vi "X10468 SLM Engine.vi"(0 "Notifier Name":string, 11 "SLM Config Info":string[](array[string])) -> ()   [LabVIEW 2018]
uses:
  X10468 Controls/X10468 SLM Notifier.ctl
  X10468 Controls/X10468 SLM Actions.ctl
  <vilib>/vision/Image Controls.llb/IMAQ Image.ctl
  X10468 Controls/X10468 SLM Last Used.ctl
panel:
  out "Holo Max":dbl
  out "Holo Min":dbl
  out "Flat File":path
  out "SLM Display":T1(plugin-control)
  out "SLM Min":u8
  out "SLM Max":u8
  in  "Mode Amounts":dbl[](array[numeric])
  in  "Holo XY Position":i32[](array[numeric])
  in  "Top Hat Radius":dbl
  in  "Holo Size (px)":i32=10 min=10 max=1000
  in  "Set Flat":bool
  in  "Flat":bool
  in  "Top Hat":bool
  in  "Vortex Direction":bool
  in  "Vortex":bool
  in  "Number of Modes":i32=1 min=1 max=32
  out "Last Error":errorcluster
  in  "Quit":bool
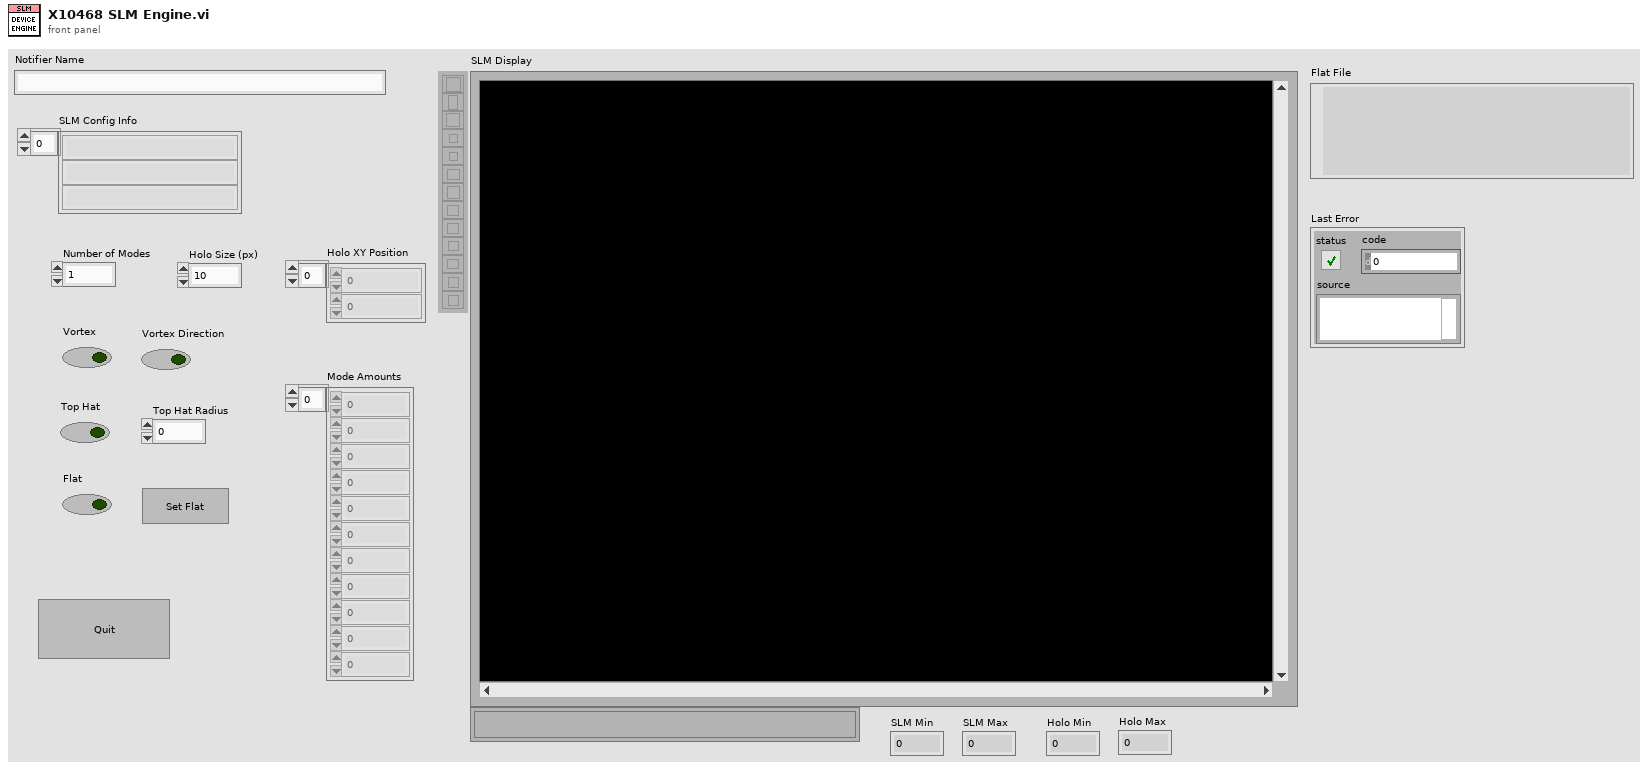
[diagram p1: front panel]
types:
  T1 = typedef "IMAQ Image.ctl" = refnum<image>
  T2 = typedef "X10468 SLM Last Used.ctl" = cluster{"Flat On?":bool, "Vortex On?":bool, "Top Hat On?":bool, "Mode Amps":dbl[], "Number of Modes":i32, "Holo Diameter (px)":i32, "Top Hat Radius":dbl, "Holo Position":i32[], "Flat File Path":string}
  T3 = typedef "X10468 SLM Actions.ctl" = enum16{"Exit Loop", "Get Settings", "Set Flat File", "Change Holo Size", "Change Num Modes", "Change Holo Position", "Change Top Hat Size", "Change Vortex Direction", "Change Mode Amounts", "Flat On/Off", "Vortex On/Off", "Top Hat On/Off", "Make Hologram", "Update SLM Display", "Quit"}
  T4 = typedef "X10468 SLM Notifier.ctl" = cluster{"SLM Actions":T3, "SLM Image":T1, "Flat On?":bool, "Vortex On?":bool, "Top Hat On?":bool, "Mode Amps":dbl[], "Number of Modes":i32, "Holo Diameter (px)":i32, "Top Hat Radius":dbl, "Holo Position":i32[], "Received?":bool, "Flat File Path":path}
  T5 = typedef "Image Type" = u32
  T6 = typedef "LVAllMonitorsDisplayTypeDef.ctl" = cluster{"Bounds":cluster{"Left":i16, "Top":i16, "Right":i16, "Bottom":i16}, "Depth":i16}[]
  T7 = cluster{"Bounds":cluster{"Left":i16, "Top":i16, "Right":i16, "Bottom":i16}, "Depth":i16}
  T8 = enum32{"Invalid", "Standard", "Closed", "Hidden", "Minimized", "Maximized"}
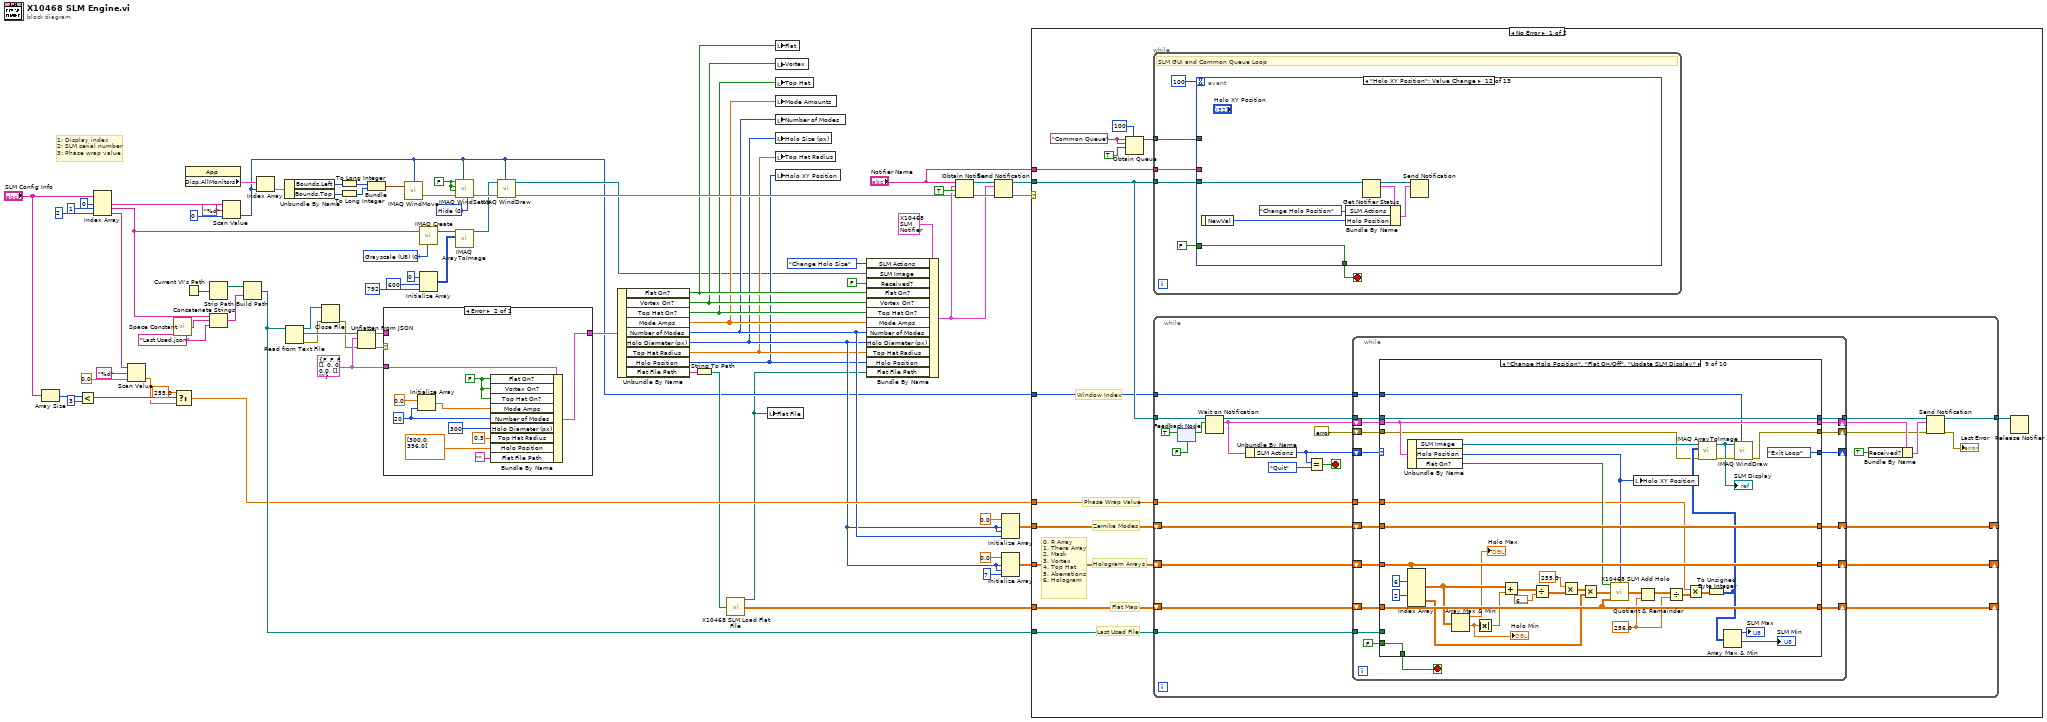
[diagram p0: block diagram]
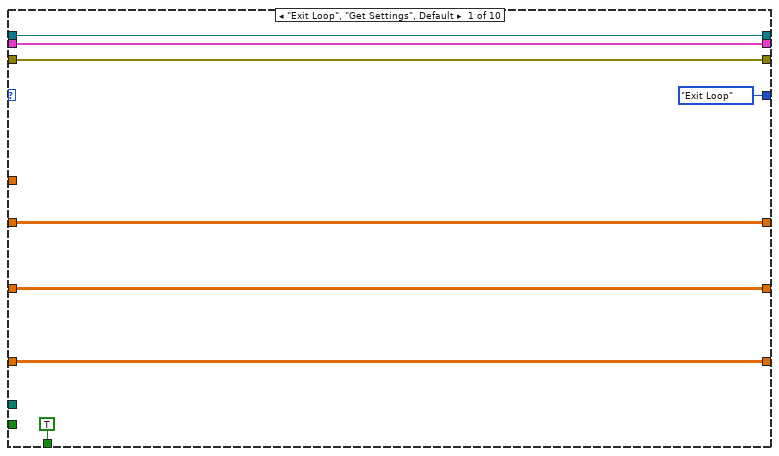
[diagram p3: hidden frame]
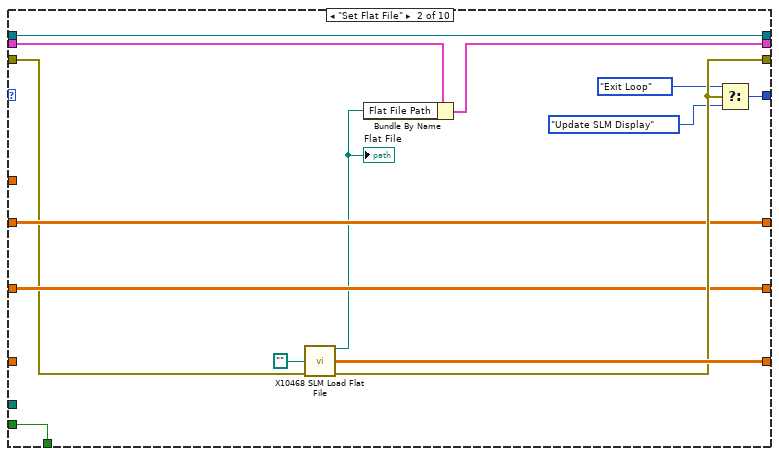
[diagram p4: hidden frame]
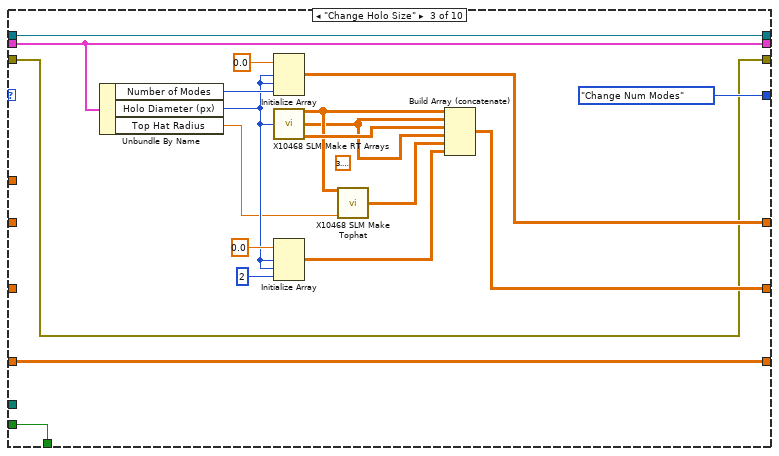
[diagram p5: hidden frame]
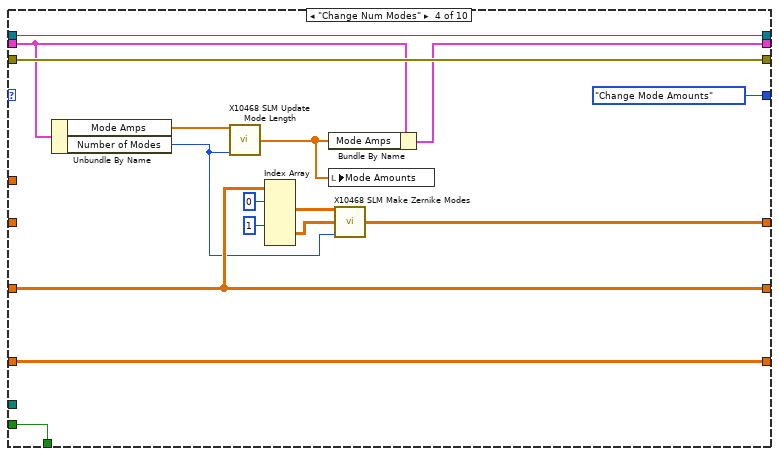
[diagram p6: hidden frame]
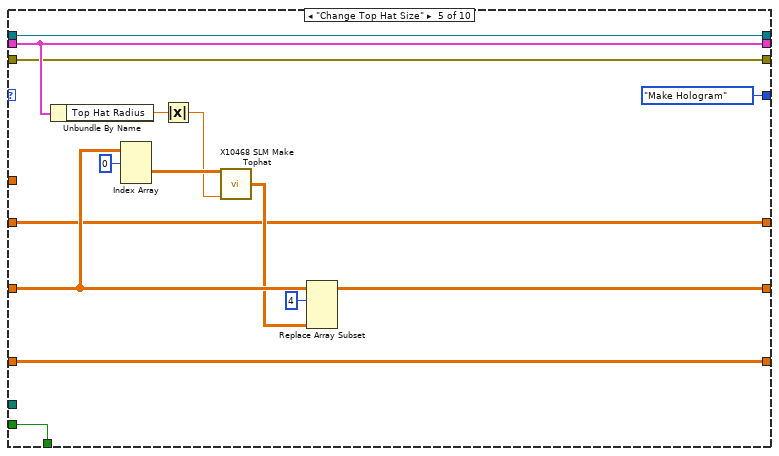
[diagram p7: hidden frame]
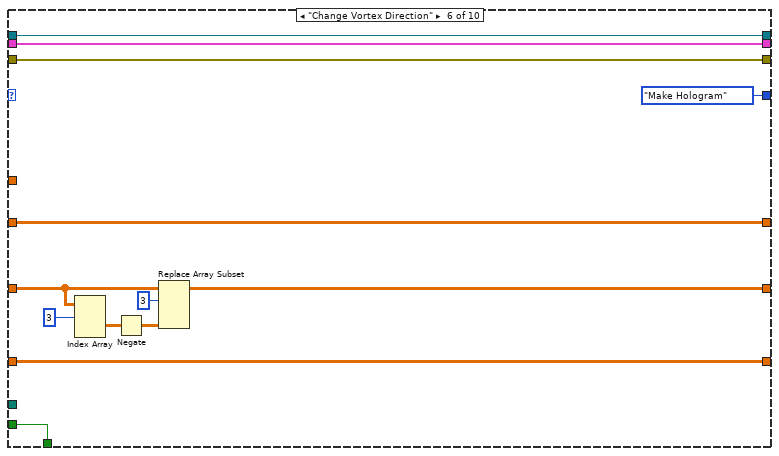
[diagram p8: hidden frame]
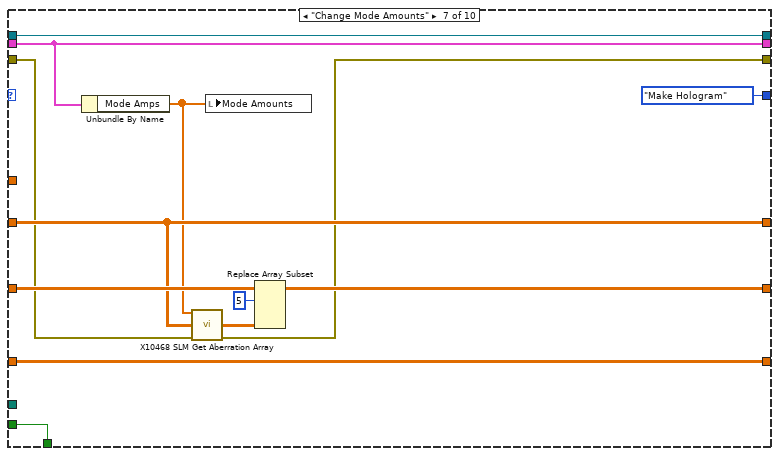
[diagram p9: hidden frame]
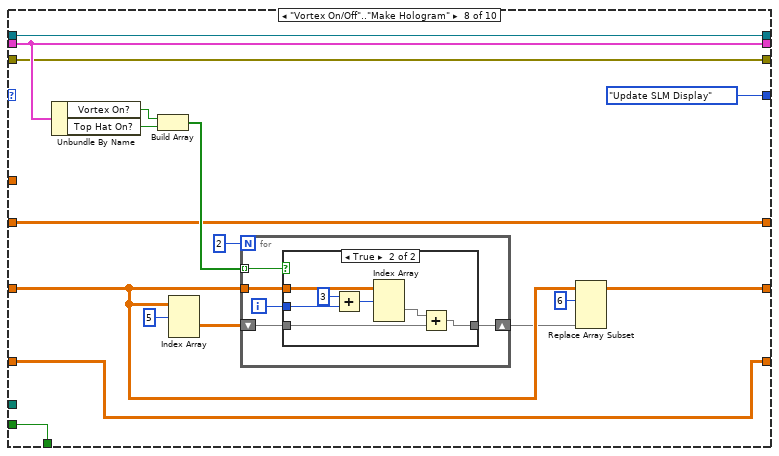
[diagram p10: hidden frame]
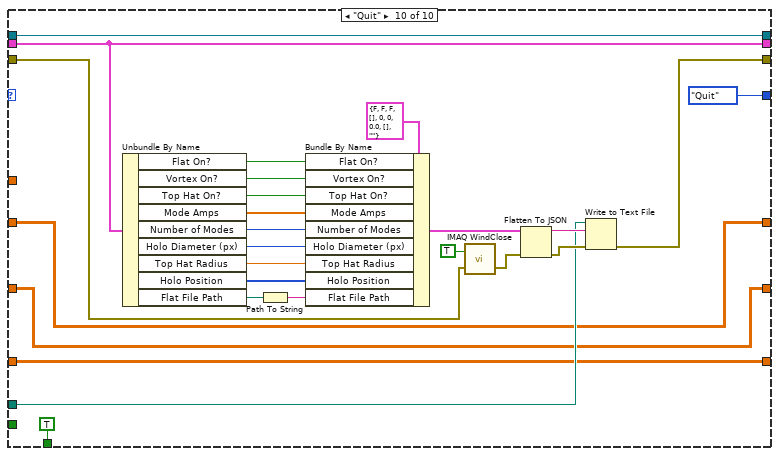
[diagram p12: hidden frame]
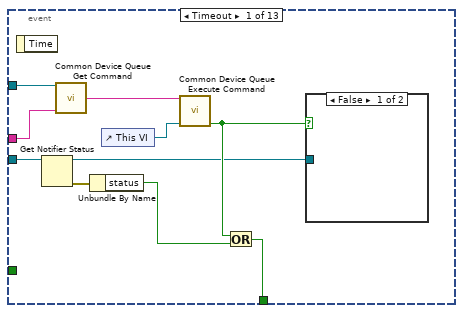
[diagram p13: hidden frame]
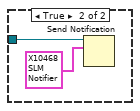
[diagram p14: hidden frame]
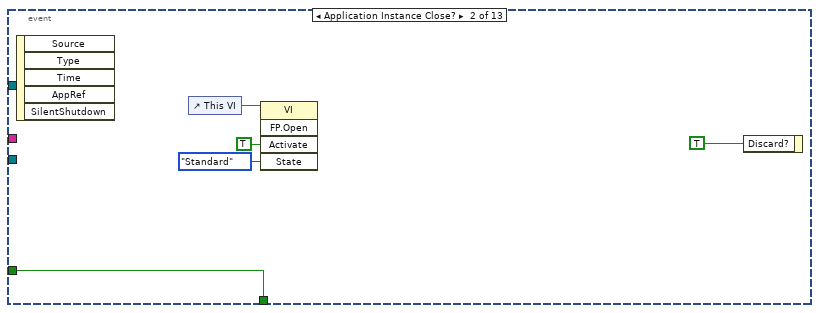
[diagram p15: hidden frame]
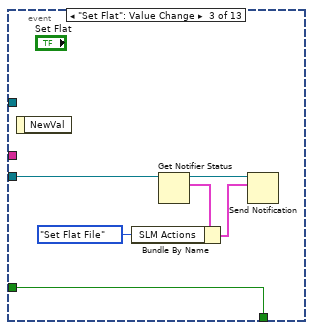
[diagram p16: hidden frame]
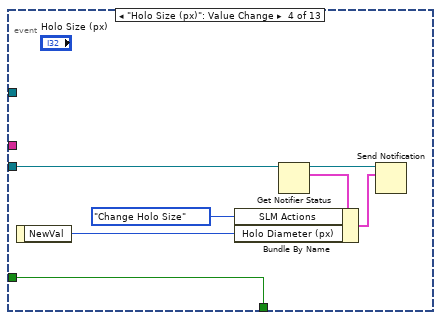
[diagram p17: hidden frame]
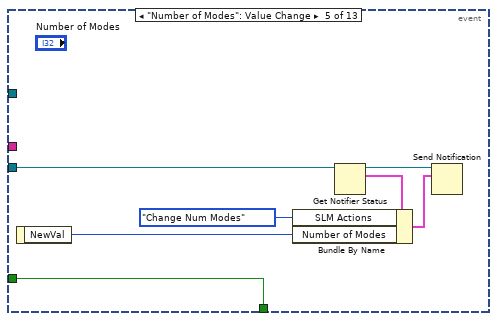
[diagram p18: hidden frame]
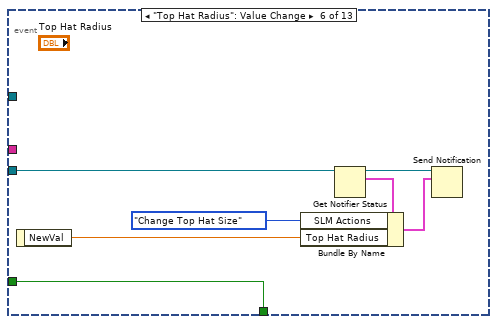
[diagram p19: hidden frame]
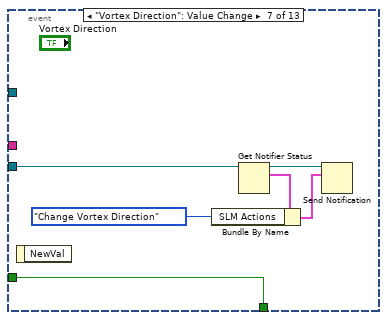
[diagram p20: hidden frame]
diagram:
  w31 = T2 {"Flat On?"=FALSE, "Vortex On?"=FALSE, "Top Hat On?"=FALSE, "Mode Amps"=[], "Number of Modes"=0, "Holo Diameter (px)"=0, "Top Hat Radius"=0.0, "Holo Position"=[], "Flat File Path"=""} ("SLM Notifier")
  w63 = 0 items=["Hide", "Show", "No change"] ("Scrollbars (No change)")
  w64 = FALSE ("Window can grow? (Yes)")
  w78 = T5 0 items=["Grayscale (U8)", "Grayscale (I16)", "Grayscale (SGL)", "Complex (CSG)", "RGB (U32)", "HSL (U32)", "RGB (U64)", "Grayscale (U16)"] ("Image Type")
  # "1: Display index\n2: SLM serial number\n3: Phase wrap value"
  n1 = Array Size(array="SLM Config Info") -> (size(s)=w43:i32)
  n2 = Less?(x=w43, y=3) -> (x < y?=w41:bool)
  n3 = Index Array(array="SLM Config Info", index #1=0 ("index"), index #2=1 ("index"), index #3=2 ("index")) -> (element #1=w72:string, element #2=w38:string, element #3=w45:string)
  n4 = Scan Value(string=w45, format string="%d", default (0 dbl)=0.0) -> (value=w40:dbl)  [unwired: 1 out]
  n5 = call <vilib>:"Space Constant.vi"() -> ("String"=w37:string)
  n6 = Select(t=255.0, s=w41, f=w40) -> (s? t:f=w23:dbl)
  n7 = property class="App"() -> ("Disp.AllMonitors"=w69:T6)  [unwired: 2 in, 2 out]
  n8 = Current VI's Path() -> (path=w75:path)
  n9 = Strip Path(path=w75) -> (stripped path=w74:path)  [unwired: 1 out]
  n10 = Concatenate Strings(w38, w37, "Last Used.json" ("string")) -> (w35:string)
  n11 = Scan Value(string=w72, format string="%d", default (0 dbl)=0) -> (value=w2:i32)  [unwired: 1 out]
  n12 = Build Path(base path=w74, name or relative path=w35) -> (appended path=w24:path)
  n13 = Index Array(array=w69, index=w2) -> (element=w68:T7)
  n14 = Unbundle By Name(w68) -> ("Bounds.Left"=w67:i16, "Bounds.Top"=w27:i16)
  n15 = Read from Text File(file (use dialog)=w24) -> (refnum out=w17:refnum<file>, text=w34:string, error out=w16:errorcluster)  [unwired: 3 in, 1 out]
  n16 = Close File(refnum=w17, error in=w16) -> (error out=w15:errorcluster)  [unwired: 1 out]
  n17 = To Long Integer(number=w27) -> (32bit integer=w26:i32)
  n18 = To Long Integer(number=w67) -> (32bit integer=w66:i32)
  n19 = Unflatten From JSON(JSON string=w34, type and defaults=w31, error in (no error)=w15) -> (value=w32:T2, error out=w33:errorcluster)  [unwired: 4 in]
  n20 = Bundle(w66, w26) -> (w65:cluster{i32, i32})  [unwired: 1 in]
  n21 = case shown="Error" w33 {
    tunnel: w32 -> [w80 _]
    tunnel: w31 -> [_ w90]
    tunnel: [w80 w83] -> w30
    frame No Error {
    }
    frame Error {
      w81 = 20 ("Number of Modes")
      w89 = FALSE ("Flat On?")
      n22 = Initialize Array(0.0 ("element"), w81) -> (w84:dbl[])
      n23 = Bundle By Name(cluster=w90, "Flat On?"=w89, "Vortex On?"=w89, "Top Hat On?"=w89, "Mode Amps"=w84, "Number of Modes"=w81, "Holo Diameter (px)"=300 ("Holo Size (px)"), "Top Hat Radius"=0.5, "Holo Position"=dbl[] [300.0, 396.0], "Flat File Path"="") -> (w83:T2)
    }
  }
  n24 = call "IMAQ WindMove"("Window Number (0...15)"=w2, "Coordinates (screen)"=w65) -> ("error out"=w62:errorcluster)  [unwired: 2 in, 2 out]
  n25 = call "IMAQ Create"("Image Name"=w38, "Image Type"=w78) -> ("New Image"=w61:T1)  [unwired: 3 in, 1 out]
  n26 = Initialize Array(u8 0 ("element"), 600 ("dimension size"), 792 ("dimension size")) -> (w57:u8[][])
  n27 = call "IMAQ ArrayToImage"("Image Pixels (U8)"=w57, "Image"=w61) -> ("Image Out"=w55:T1)  [unwired: 8 in, 1 out]
  n28 = call "IMAQ WindSetup"("Scrollbars (No change)"=w63, "Window Number (0...15)"=w2, "error in (no error)"=w62, "Window has title bar? (Yes)"=w64, "Window can close? (Yes)"=w64, "Window can grow? (Yes)"=w64) -> ("error out"=w56:errorcluster)  [unwired: 1 in, 4 out]
  n29 = call "IMAQ WindDraw"("Window Number (0...15)"=w2, "error in (no error)"=w56, "Image"=w55) -> ("error out"=w28:errorcluster, "Image Out (duplicate)"=w3:T1)  [unwired: 3 in, 4 out]
  n30 = Unbundle By Name(w30) -> ("Flat On?"=w12:bool, "Vortex On?"=w11:bool, "Top Hat On?"=w10:bool, "Mode Amps"=w9:dbl[], "Number of Modes"=w8:i32, "Holo Diameter (px)"=w7:i32, "Top Hat Radius"=w6:dbl, "Holo Position"=w5:i32[], "Flat File Path"=w22:string)
  n31 = String To Path(string=w22) -> (path=w4:path)
  n32 = call "X10468 SLM Load Flat File.vi"("Flat File Path"=w4) -> ("Selected File"=w1:path, "SLM Flat Map"=w21:dbl[][])  [unwired: 12 in, 1 out]
  n33 = local write "Flat File"(w1) -> ()
  n34 = local write "Flat"(w12) -> ()
  n35 = local write "Vortex"(w11) -> ()
  n36 = local write "Top Hat"(w10) -> ()
  n37 = local write "Mode Amounts"(w9) -> ()
  n38 = local write "Number of Modes"(w8) -> ()
  n39 = local write "Holo Size (px)"(w7) -> ()
  n40 = local write "Top Hat Radius"(w6) -> ()
  n41 = local write "Holo XY Position"(w5) -> ()
  n42 = Bundle By Name(cluster=T4 {"SLM Actions"=enum."Exit Loop", "SLM Image"=refnum, "Flat On?"=FALSE, "Vortex On?"=FALSE, "Top Hat On?"=FALSE, "Mode Amps"=[], "Number of Modes"=0, "Holo Diameter (px)"=0, "Top Hat Radius"=0.0, "Holo Position"=[], "Received?"=FALSE, "Flat File Path"=path ""} ("SLM Notifier"), "SLM Actions"=X10468_SLM_Actions."Change Holo Size", "SLM Image"=w3, "Received?"=FALSE, "Flat On?"=w12, "Vortex On?"=w11, "Top Hat On?"=w10, "Mode Amps"=w9, "Number of Modes"=w8, "Holo Diameter (px)"=w7, "Top Hat Radius"=w6, "Holo Position"=w5, "Flat File Path"=w1) -> (w49:T4)
  n43 = Obtain Notifier(name (unnamed)="Notifier Name", notification data type=w49, create if not found? (T)=TRUE, error in (no error)=w28) -> (notifier out=w52:refnum<notifier>, error out=w50:errorcluster)  [unwired: 1 out]
  n44 = Send Notification(notification=w49, notifier=w52, error in (no error)=w50) -> (notifier out=w51:refnum<notifier>, error out=w25:errorcluster)
  n45 = Initialize Array(0.0 ("element"), w7, w7, w8) -> (w13:dbl[][][])
  n46 = Initialize Array(0.0 ("element"), w7, w7, 7 ("dimension size")) -> (w18:dbl[][][])
  n47 = case shown="No Error" w25 {
    tunnel: w51 -> [w98 w438]
    tunnel: "Notifier Name" -> [w99 _]
    tunnel: w24 -> [w96 _]
    tunnel: w23 -> [w93 _]
    tunnel: w21 -> [w95 _]
    tunnel: w18 -> [w94 _]
    tunnel: w13 -> [w92 _]
    tunnel: w2 -> [w91 _]
    frame No Error {
      w103 = "Common Queue" ("Unique Notifier Name")
      # "Window Index"
      # "Zernike Modes"
      # "Last Used File"
      # "Phase Wrap Value"
      # "0. R Array\n1. Thera Array\n2. Mask\n3. Vortex\n4. Top Hat\n5. Aberrations\n6. Hologram"
      # "Hologram Arrays"
      # "Flat Map"
      n48 = Obtain Queue(max queue size (-1, unlimited)=100, name (unnamed)=w103, element data type=w103, create if not found? (T)=TRUE) -> (queue out=w100:refnum<queue>)  [unwired: 1 in, 2 out]
      n49 = while {
        tunnel: w100 -> [w344]
        tunnel: w99 -> [w342]
        tunnel: w98 -> [w343]
        stop <- w341 stop-if-true
        # "SLM GUI and Common Queue Loop"
        n50 = event shown="[11] \"Holo XY Position\": Value Change" {
          selector: _ -> [_ _ _ _ _ _ _ _ _ _ _ _ _]
          dyn-events: _ -> [_ _ _ _ _ _ _ _ _ _ _ _ _]
          timeout: 100 -> [_ _ _ _ _ _ _ _ _ _ _ _ _]
          tunnel: w344 -> [w349 _ _ _ _ _ _ _ _ _ _ _ w437]
          tunnel: w343 -> [w348 _ w368 w375 w382 w389 w395 w402 w409 w416 w423 w430 w436]
          tunnel: w342 -> [w347 _ _ _ _ _ _ _ _ _ _ _ _]
          tunnel: [w346 w362 w363 w370 w377 w384 w390 w397 w405 w412 w419 w426 w432] -> w341
          tunnel: FALSE -> [_ w362 w363 w370 w377 w384 w390 w397 w405 w412 w419 w426 _]
          event Timeout {
            n51 = event-data() -> ()  [unwired: 1 in, 1 out]
            n52 = Get Notifier Status(notifier=w348) -> (notifier out=w350:refnum<notifier>, error out=w355:errorcluster)  [unwired: 1 in, 3 out]
            n53 = call "Common Device Queue Get Command.vi"("Common Queue"=w349, "Notifier Name"=w347) -> ("Command"=w354:string)  [unwired: 12 in, 1 out]
            n54 = Unbundle By Name(w355) -> ("status"=w352:bool)
            n55 = control-ref of="This VI"() -> (w353:refnum<vi>)
            n56 = call "Common Device Queue Execute Command.vi"("Common Command"=w354, "VI Refnum"=w353) -> ("Quit?"=w351:bool)  [unwired: 12 in, 1 out]
            n57 = Or(x=w351, y=w352) -> (x .or. y?=w346:bool)
            n58 = case shown="False" w351 {
              tunnel: w350 -> [_ w357]
              frame False {
              }
              frame True {
                n59 = Send Notification(notification=T4 {"SLM Actions"=enum."Quit", "SLM Image"=refnum, "Flat On?"=FALSE, "Vortex On?"=FALSE, "Top Hat On?"=FALSE, "Mode Amps"=[], "Number of Modes"=0, "Holo Diameter (px)"=0, "Top Hat Radius"=0.0, "Holo Position"=[], "Received?"=FALSE, "Flat File Path"=path ""} ("SLM Notifier"), notifier=w357) -> ()  [unwired: 1 in, 2 out]
              }
            }
          }
          event Application Instance Close? {
            n60 = event-data() -> ()  [unwired: 1 in, 5 out]
            n61 = control-ref of="This VI"() -> (w359:refnum<vi>)
            n62 = invoke class="VI" method="FP.Open"(reference=w359, "Activate"=TRUE ("Activate?"), "State"=T8."Standard") -> ()  [unwired: 2 in, 5 out]
            n63 = event-data("Discard?"=TRUE) -> ()  [unwired: 1 in, 1 out]
          }
          event "Set Flat": Value Change {
            n64 = event-data() -> ()  [unwired: 1 in, 1 out]
            n65 = Get Notifier Status(notifier=w368) -> (notifier out=w367:refnum<notifier>, current notification=w366:T4)  [unwired: 1 in, 3 out]
            n66 = Bundle By Name(cluster=w366, "SLM Actions"=X10468_SLM_Actions."Set Flat File") -> (w364:T4)
            n67 = Send Notification(notification=w364, notifier=w367) -> ()  [unwired: 1 in, 2 out]
          }
          event "Holo Size (px)": Value Change {
            n68 = event-data() -> ("NewVal"=w369:i32)  [unwired: 1 in]
            n69 = Get Notifier Status(notifier=w375) -> (notifier out=w374:refnum<notifier>, current notification=w373:T4)  [unwired: 1 in, 3 out]
            n70 = Bundle By Name(cluster=w373, "SLM Actions"=X10468_SLM_Actions."Change Holo Size", "Holo Diameter (px)"=w369) -> (w371:T4)
            n71 = Send Notification(notification=w371, notifier=w374) -> ()  [unwired: 1 in, 2 out]
          }
          event "Number of Modes": Value Change {
            n72 = event-data() -> ("NewVal"=w376:i32)  [unwired: 1 in]
            n73 = Get Notifier Status(notifier=w382) -> (notifier out=w381:refnum<notifier>, current notification=w380:T4)  [unwired: 1 in, 3 out]
            n74 = Bundle By Name(cluster=w380, "SLM Actions"=X10468_SLM_Actions."Change Num Modes", "Number of Modes"=w376) -> (w378:T4)
            n75 = Send Notification(notification=w378, notifier=w381) -> ()  [unwired: 1 in, 2 out]
          }
          event "Top Hat Radius": Value Change {
            n76 = event-data() -> ("NewVal"=w383:dbl)  [unwired: 1 in]
            n77 = Get Notifier Status(notifier=w389) -> (notifier out=w388:refnum<notifier>, current notification=w387:T4)  [unwired: 1 in, 3 out]
            n78 = Bundle By Name(cluster=w387, "SLM Actions"=X10468_SLM_Actions."Change Top Hat Size", "Top Hat Radius"=w383) -> (w385:T4)
            n79 = Send Notification(notification=w385, notifier=w388) -> ()  [unwired: 1 in, 2 out]
          }
          event "Vortex Direction": Value Change {
            n80 = event-data() -> ()  [unwired: 1 in, 1 out]
            n81 = Get Notifier Status(notifier=w395) -> (notifier out=w394:refnum<notifier>, current notification=w393:T4)  [unwired: 1 in, 3 out]
            n82 = Bundle By Name(cluster=w393, "SLM Actions"=X10468_SLM_Actions."Change Vortex Direction") -> (w391:T4)
            n83 = Send Notification(notification=w391, notifier=w394) -> ()  [unwired: 1 in, 2 out]
          }
          event "Mode Amounts": Value Change {
            n84 = event-data() -> ("NewVal"=w396:dbl[])  [unwired: 1 in]
            n85 = Get Notifier Status(notifier=w402) -> (notifier out=w401:refnum<notifier>, current notification=w400:T4)  [unwired: 1 in, 3 out]
            n86 = Bundle By Name(cluster=w400, "SLM Actions"=X10468_SLM_Actions."Change Mode Amounts", "Mode Amps"=w396) -> (w398:T4)
            n87 = Send Notification(notification=w398, notifier=w401) -> ()  [unwired: 1 in, 2 out]
          }
          event "Vortex": Value Change {
            n88 = event-data() -> ("NewVal"=w403:bool)  [unwired: 1 in]
            n89 = Get Notifier Status(notifier=w409) -> (notifier out=w408:refnum<notifier>, current notification=w407:T4)  [unwired: 1 in, 3 out]
            n90 = Bundle By Name(cluster=w407, "SLM Actions"=X10468_SLM_Actions."Vortex On/Off", "Vortex On?"=w403) -> (w406:T4)
            n91 = Send Notification(notification=w406, notifier=w408) -> ()  [unwired: 1 in, 2 out]
          }
          event "Top Hat": Value Change {
            n92 = event-data() -> ("NewVal"=w410:bool)  [unwired: 1 in]
            n93 = Get Notifier Status(notifier=w416) -> (notifier out=w415:refnum<notifier>, current notification=w414:T4)  [unwired: 1 in, 3 out]
            n94 = Bundle By Name(cluster=w414, "SLM Actions"=X10468_SLM_Actions."Top Hat On/Off", "Top Hat On?"=w410) -> (w413:T4)
            n95 = Send Notification(notification=w413, notifier=w415) -> ()  [unwired: 1 in, 2 out]
          }
          event "Flat": Value Change {
            n96 = event-data() -> ("NewVal"=w417:bool)  [unwired: 1 in]
            n97 = Get Notifier Status(notifier=w423) -> (notifier out=w422:refnum<notifier>, current notification=w421:T4)  [unwired: 1 in, 3 out]
            n98 = Bundle By Name(cluster=w421, "SLM Actions"=X10468_SLM_Actions."Flat On/Off", "Flat On?"=w417) -> (w420:T4)
            n99 = Send Notification(notification=w420, notifier=w422) -> ()  [unwired: 1 in, 2 out]
          }
          event "Holo XY Position": Value Change {
            n100 = event-data() -> ("NewVal"=w424:i32[])  [unwired: 1 in]
            n101 = Get Notifier Status(notifier=w430) -> (notifier out=w429:refnum<notifier>, current notification=w428:T4)  [unwired: 1 in, 3 out]
            n102 = Bundle By Name(cluster=w428, "SLM Actions"=X10468_SLM_Actions."Change Holo Position", "Holo Position"=w424) -> (w427:T4)
            n103 = Send Notification(notification=w427, notifier=w429) -> ()  [unwired: 1 in, 2 out]
          }
          event "Quit": Value Change {
            n104 = event-data() -> ("NewVal"=w432:bool)  [unwired: 1 in]
            n105 = Release Queue(queue=w437) -> ()  [unwired: 2 in, 3 out]
            n106 = Get Notifier Status(notifier=w436) -> (notifier out=w435:refnum<notifier>, current notification=w434:T4)  [unwired: 1 in, 3 out]
            n107 = Bundle By Name(cluster=w434, "SLM Actions"=X10468_SLM_Actions."Quit") -> (w433:T4)
            n108 = Send Notification(notification=w433, notifier=w435) -> ()  [unwired: 1 in, 2 out]
          }
        }
      }
      n109 = while {
        tunnel: w98 -> [w129]
        tunnel: [w123] -> w97
        tunnel: w96 -> [w121]
        shift-right: [w119] -> _
        shift-left: w95 -> [w120]
        shift-right: [w114] -> _
        shift-left: w94 -> [w118]
        tunnel: w93 -> [w115]
        shift-right: [w116] -> _
        shift-left: w92 -> [w117]
        tunnel: w91 -> [w110]
        stop <- w128 stop-if-true
        n110 = feedback #1(FALSE ("ignore previous (F)")) -> (w112:bool)
        n111 = feedback-in #1(TRUE ("ignore previous (F)")) -> ()
        n112 = Wait on Notification(notifier=w129, ignore previous (F)=w112) -> (notifier out=w126:refnum<notifier>, notification=w125:T4)  [unwired: 2 in, 2 out]
        n113 = Unbundle By Name(w125) -> ("SLM Actions"=w127:T3)
        n114 = Equal?(x=w127, y=X10468_SLM_Actions."Quit") -> (x = y?=w128:bool)
        n115 = while {
          tunnel: w121 -> [w142]
          shift-right: [w140] -> w119
          shift-left: w120 -> [w141]
          tunnel: w126 -> [w147]
          tunnel: [w145] -> w106
          shift-right: [w136] -> w116
          shift-left: w117 -> [w137]
          shift-right: [w138] -> w114
          shift-left: w118 -> [w139]
          shift-right: [w132] -> _
          shift-left: w127 -> [w148]
          tunnel: w115 -> [w135]
          tunnel: w110 -> [w131]
          shift-right: [w143] -> w104
          shift-left: errorcluster {"status"=FALSE, "code"=0, "source"=""} ("error out") -> [w130]
          shift-right: [w144] -> w108
          shift-left: w125 -> [w146]
          stop <- w133 stop-if-true
          n116 = case shown="\"Change Holo Position\", \"Flat On/Off\", \"Update SLM Display\"" w148 {
            tunnel: w147 -> [w156 w170 w188 w205 w220 w233 w246 w263 w313 w339]
            tunnel: w146 -> [w155 w160 w187 w192 w210 w232 w245 w251 w309 w338]
            tunnel: [w156 w170 w188 w205 w220 w233 w246 w263 w313 w339] -> w145
            tunnel: [w155 w159 w187 w191 w210 w232 w245 w251 w309 w338] -> w144
            tunnel: [w149 w168 w171 w195 w206 w221 w238 w247 w278 w324] -> w143
            tunnel: w142 -> [_ _ _ _ _ _ _ _ _ w325]
            tunnel: w141 -> [w154 _ w189 w204 w211 w225 w239 w256 w303 w321]
            tunnel: [w154 w169 w189 w204 w211 w225 w239 w256 w303 w321] -> w140
            tunnel: w139 -> [w151 w162 _ w202 w216 w226 w244 w254 w305 w318]
            tunnel: [w151 w162 w176 w202 w213 w227 w240 w253 w305 w318] -> w138
            tunnel: w137 -> [w152 w163 _ _ w212 w224 w241 w255 w312 w317]
            tunnel: [w152 w163 w184 w203 w212 w224 w241 w255 w312 w317] -> w136
            tunnel: w135 -> [_ _ _ _ _ _ _ _ w283 _]
            tunnel: FALSE -> [_ w164 w175 w201 w208 w222 w236 w249 w311 _]
            tunnel: [TRUE w164 w175 w201 w208 w222 w236 w249 w311 TRUE] -> w133
            tunnel: [X10468_SLM_Actions."Exit Loop" ("y") w166 X10468_SLM_Actions."Change Num Modes" ("y") X10468_SLM_Actions."Change Mode Amounts" ("y") X10468_SLM_Actions."Make Hologram" ("y") X10468_SLM_Actions."Make Hologram" ("y") X10468_SLM_Actions."Make Hologram" ("y") X10468_SLM_Actions."Update SLM Display" ("y") X10468_SLM_Actions."Exit Loop" ("y") X10468_SLM_Actions."Quit" ("y")] -> w132
            tunnel: w131 -> [_ _ _ _ _ _ _ _ w306 _]
            tunnel: w130 -> [w149 w157 w171 w195 w206 w221 w235 w247 w279 w314]
            frame "Exit Loop", "Get Settings", Default {
            }
            frame "Set Flat File" {
              n117 = call "X10468 SLM Load Flat File.vi"("Flat File Path"=path "", "Error In"=w157) -> ("Selected File"=w158:path, "SLM Flat Map"=w169:dbl[][], "Error Out"=w168:errorcluster)  [unwired: 11 in]
              "Flat File" <- w158
              n118 = Bundle By Name(cluster=w160, "Flat File Path"=w158) -> (w159:T4)
              n119 = Select(t=X10468_SLM_Actions."Exit Loop" ("y"), s=w168, f=X10468_SLM_Actions."Update SLM Display" ("y")) -> (s? t:f=w166:T3)
            }
            frame "Change Holo Size" {
              (unwired) 3.141592653589793
              n120 = Unbundle By Name(w187) -> ("Number of Modes"=w185:i32, "Holo Diameter (px)"=w182:i32, "Top Hat Radius"=w178:dbl)
              n121 = Initialize Array(0.0 ("element"), w182, w182, w185) -> (w184:dbl[][][])
              n122 = call "X10468 SLM Make RT Arrays.vi"("Holo Diameter (px)"=w182) -> ("R Array"=w180:dbl[][], "Theta Array"=w172:dbl[][], "Mask Array"=w181:dbl[][])  [unwired: 12 in]
              n123 = Initialize Array(0.0 ("element"), w182, w182, 2 ("dimension size")) -> (w177:dbl[][][])
              n124 = call "X10468 SLM Make Tophat.vi"("R Array"=w180, "Normalized Radius"=w178) -> ("Tophat Holo"=w179:dbl[][])  [unwired: 13 in]
              n125 = Build Array (concatenate)(w180, w172, w181, w172, w179, w177) -> (w176:dbl[][][])
            }
            frame "Change Num Modes" {
              n126 = Unbundle By Name(w192) -> ("Mode Amps"=w193:dbl[], "Number of Modes"=w194:i32)
              n127 = call "X10468 SLM Update Mode Length.vi"("Mode Amp"=w193, "Number of Modes"=w194) -> ("Adjusted Mode Amps"=w190:dbl[])  [unwired: 13 in]
              n128 = Index Array(array=w202, index (dim 0) #1=0 ("index (page)"), index (dim 0) #2=1 ("index (page)")) -> (element #1=w197:dbl[][], element #2=w196:dbl[][])  [unwired: 4 in]
              n129 = Bundle By Name(cluster=w192, "Mode Amps"=w190) -> (w191:T4)
              n130 = local write "Mode Amounts"(w190) -> ()
              n131 = call "X10468 SLM Make Zernike Modes.vi"("R Array"=w197, "Theta Array"=w196, "Number of Modes"=w194) -> ("Zernike Array"=w203:dbl[][][])  [unwired: 12 in]
            }
            frame "Change Top Hat Size" {
              n132 = Unbundle By Name(w210) -> ("Top Hat Radius"=w217:dbl)
              n133 = Index Array(array=w216, index (dim 0)=0 ("index (page)")) -> (element=w218:dbl[][])  [unwired: 2 in]
              n134 = Absolute Value(x=w217) -> (abs(x)=w207:dbl)
              n135 = call "X10468 SLM Make Tophat.vi"("R Array"=w218, "Normalized Radius"=w207) -> ("Tophat Holo"=w214:dbl[][])  [unwired: 13 in]
              n136 = Replace Array Subset(array=w216, new element=w214, index (dim 0)=4 ("index (page)")) -> (w213:dbl[][][])  [unwired: 2 in]
            }
            frame "Change Vortex Direction" {
              n137 = Index Array(array=w226, index (dim 0)=3 ("index (page)")) -> (element=w229:dbl[][])  [unwired: 2 in]
              n138 = Negate(x=w229) -> (-x=w228:dbl[][])
              n139 = Replace Array Subset(array=w226, new element=w228, index (dim 0)=3 ("index (page)")) -> (w227:dbl[][][])  [unwired: 2 in]
            }
            frame "Change Mode Amounts" {
              n140 = Unbundle By Name(w245) -> ("Mode Amps"=w234:dbl[])
              n141 = call "X10468 SLM Get Aberration Array.vi"("Mode Amps"=w234, "Zernike Modes"=w241, "Error In"=w235) -> ("Aberration Array"=w242:dbl[][], "Error Out"=w238:errorcluster)  [unwired: 11 in]
              n142 = local write "Mode Amounts"(w234) -> ()
              n143 = Replace Array Subset(array=w244, new element=w242, index (dim 0)=5 ("index (page)")) -> (w240:dbl[][][])  [unwired: 2 in]
            }
            frame "Vortex On/Off".."Make Hologram" {
              n144 = Unbundle By Name(w251) -> ("Vortex On?"=w260:bool, "Top Hat On?"=w259:bool)
              n145 = Build Array(w260, w259) -> (w257:bool[])
              n146 = Index Array(array=w254, index (dim 0)=5 ("index (page)")) -> (element=w261:dbl[][])  [unwired: 2 in]
              n147 = for {
                N: 2 -> [_]
                shift-right: [w267] -> w248
                shift-left: w261 -> [w268]
                tunnel: w254 -> [w266]
                tunnel: w257 -> [w264] mode=indexing
                i -> [w265]
                n148 = case shown="True" w264 {
                  tunnel: w268 -> [w269 w270]
                  tunnel: [w269 w271] -> w267
                  tunnel: w266 -> [_ w275]
                  tunnel: w265 -> [_ w273]
                  frame False {
                  }
                  frame True {
                    n149 = Add(x=3, y=w273) -> (x+y=w274:i32)
                    n150 = Index Array(array=w275, index (dim 0)=w274) -> (element=w272:dbl[][])  [unwired: 2 in]
                    n151 = Add(x=w272, y=w270) -> (x+y=w271:dbl[][])
                  }
                }
              }
              n152 = Replace Array Subset(array=w254, new element=w248, index (dim 0)=6 ("index (page)")) -> (w253:dbl[][][])  [unwired: 2 in]
            }
            frame "Change Holo Position", "Flat On/Off", "Update SLM Display" {
              w280 = 256.0
              n153 = Unbundle By Name(w309) -> ("SLM Image"=w308:T1, "Holo Position"=w277:i32[], "Flat On?"=w292:bool)
              n154 = Index Array(array=w305, index (dim 0) #1=6 ("index (page)"), index (dim 0) #2=2 ("index (page)")) -> (element #1=w288:dbl[][], element #2=w295:dbl[][])  [unwired: 4 in]
              n155 = Array Max & Min(array=w288) -> (max value=→"Holo Max":dbl, min value=w287:dbl)  [unwired: 2 out]
              "Holo Min" <- w287
              n156 = Absolute Value(x=w287) -> (abs(x)=w299:dbl)
              n157 = Add(x=w288, y=w299) -> (x+y=w298:dbl[][])
              n158 = Divide(x=w298, y=6.283185307179586) -> (x/y=w301:dbl[][])
              n159 = Multiply(x=255.0, y=w301) -> (x*y=w297:dbl[][])
              n160 = Multiply(x=w297, y=w295) -> (x*y=w294:dbl[][])
              n161 = call "X10468 SLM Add Holo.vi"("Flat On?"=w292, "Holo Position"=w277, "Holo Array"=w294, "Flat Map"=w303) -> ("Merged Flat Holo"=w293:dbl[][])  [unwired: 11 in]
              n162 = local write "Holo XY Position"(w277) -> ()
              n163 = Quotient & Remainder(x=w293, y=w280) -> (x-y*floor(x/y)=w285:dbl[][])  [unwired: 1 out]
              n164 = Divide(x=w285, y=w280) -> (x/y=w284:dbl[][])
              n165 = Multiply(x=w283, y=w284) -> (x*y=w282:dbl[][])
              n166 = To Unsigned Byte Integer(number=w282) -> (unsigned 8bit integer=w281:u8[][])
              n167 = call "IMAQ ArrayToImage"("error in (no error)"=w279, "Image Pixels (U8)"=w281, "Image"=w308) -> ("error out"=w307:errorcluster, "Image Out"=w289:T1)  [unwired: 7 in]
              "SLM Display" <- w289
              n168 = Array Max & Min(array=w281) -> (max value=→"SLM Max":u8, min value=→"SLM Min":u8)  [unwired: 2 out]
              n169 = call "IMAQ WindDraw"("Window Number (0...15)"=w306, "error in (no error)"=w307, "Image"=w289) -> ("error out"=w278:errorcluster)  [unwired: 7 in, 1 out]
            }
            frame "Quit" {
              n170 = Unbundle By Name(w338) -> ("Flat On?"=w336:bool, "Vortex On?"=w335:bool, "Top Hat On?"=w334:bool, "Mode Amps"=w333:dbl[], "Number of Modes"=w332:i32, "Holo Diameter (px)"=w331:i32, "Top Hat Radius"=w330:dbl, "Holo Position"=w329:i32[], "Flat File Path"=w323:path)
              n171 = Path To String(path=w323) -> (string=w322:string)
              n172 = Bundle By Name(cluster=T2 {"Flat On?"=FALSE, "Vortex On?"=FALSE, "Top Hat On?"=FALSE, "Mode Amps"=[], "Number of Modes"=0, "Holo Diameter (px)"=0, "Top Hat Radius"=0.0, "Holo Position"=[], "Flat File Path"=""} ("SLM Notifier"), "Flat On?"=w336, "Vortex On?"=w335, "Top Hat On?"=w334, "Mode Amps"=w333, "Number of Modes"=w332, "Holo Diameter (px)"=w331, "Top Hat Radius"=w330, "Holo Position"=w329, "Flat File Path"=w322) -> (w328:T2)
              n173 = call "IMAQ WindClose"("Close All Windows (False)"=TRUE, "error in (no error)"=w314) -> ("error out"=w315:errorcluster)  [unwired: 4 in]
              n174 = Flatten To JSON(anything=w328, error in (no error)=w315) -> (JSON string=w327:string, 11:w326:errorcluster)  [unwired: 1 in]
              n175 = Write to Text File(file (use dialog)=w325, text=w327, error in=w326) -> (error out=w324:errorcluster)  [unwired: 1 in, 2 out]
            }
          }
        }
        n176 = Bundle By Name(cluster=w108, "Received?"=TRUE) -> (w105:T4)
        n177 = Send Notification(notification=w105, notifier=w106, error in (no error)=w104) -> (notifier out=w123:refnum<notifier>, error out=→"Last Error":errorcluster)
      }
      n178 = Release Notifier(notifier=w97) -> ()  [unwired: 2 in, 3 out]
    }
    frame Error {
      n179 = One Button Dialog(message="SLM startup error.") -> ()  [unwired: 1 in, 1 out]
      n180 = Release Notifier(notifier=w438) -> ()  [unwired: 2 in, 3 out]
    }
  }
